vi "Read Power.vi"(8 "error in (no error)":errorcluster, 11 "VISA resource name":refnum<visa-resource-name>) -> (0 "error out":errorcluster, 2 "Power (watts)":dbl, 3 "VISA resource name out":refnum<visa-resource-name>)   [LabVIEW 2012, in "Fluke 5080.lvlib"]
doc: "Returns the equivalent real power for AC and DC Power outputs, based on the voltage and current settings, and power factor (AC only)."
uses:
  <instrlib>/Fluke 5080/Fluke 5080.lvlib
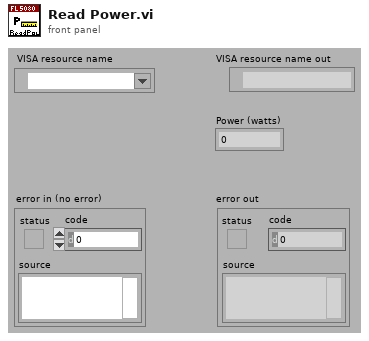
[diagram p1: front panel]
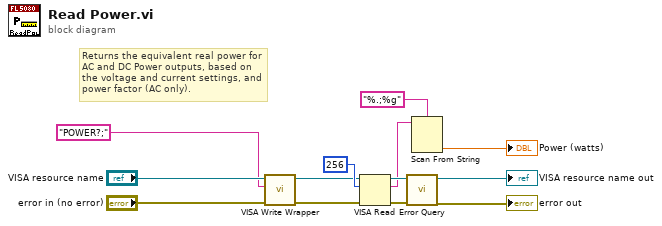
[diagram p0: block diagram]
diagram:
  # "Returns the equivalent real power for \nAC and DC Power outputs, based on \nthe voltage and current settings, and \npower factor (AC only)."
  n1 = call <instrlib>:"VISA Write Wrapper.vi"("error in (no error)"="error in (no error)", "Write Buffer"="POWER?;", "VISA resource name"="VISA resource name") -> ("error out"=w4:errorcluster, "VISA resource name out"=w5:refnum<visa-resource-name>)  [unwired: 7 out]
  n2 = VISA Read(VISA resource name=w5, byte count=u32 256, error in (no error)=w4) -> (VISA resource name out=w10:refnum<visa-resource-name>, read buffer=w8:string, error out=w9:errorcluster)  [unwired: 1 out]
  n3 = call <instrlib>:"Error Query.vi"("error in (no error)"=w9, "VISA resource name"=w10) -> ("error out"=→"error out":errorcluster, "VISA resource name out"=→"VISA resource name out":refnum<visa-resource-name>)  [unwired: 8 out]
  n4 = Scan From String(format string="%.;%g", input string=w8) -> (output 1=→"Power (watts)":dbl)  [unwired: 2 in, 4 out]
